vi "SPI API Rack FPGA Modular.vi"() -> ()   [LabVIEW 2014]
uses:
  <userlib>/_NI SPI IP/FPGA/Controllers/Public/Transfer Settings.ctl
  <vilib>/Platform/TimedLoop/XDataNode/timing_clust.ctl
  <vilib>/Platform/TimedLoop/XDataNode/nitl_modes.ctl
  <vilib>/Platform/TimedLoop/XDataNode/wakeup.ctl
  <vilib>/SPI API/SPIAPI/DIO/SPI Digital IO Lines.ctl
  Source/Shared/SPI Utility/CS Bits.ctl
  <vilib>/rvi/Emulation/niFpgaGetClockAttributes.vi
  <vilib>/rvi/Emulation/niFpgaSctlEmulationGetInTimedLoop.vi
  <vilib>/rvi/Emulation/niFpgaEmulationReportErrorSimple.vi
  <vilib>/rvi/Emulation/niFpgaCriticalErrorInLSC.vi
  <vilib>/rvi/interface/RandomDataEmulation/niFpgaRandomDataHandleErrors.vi
  <vilib>/rvi/eio/common/nirviEmuTemplateMethod_errors.vi
  <vilib>/Platform/TimedLoop/XDataNode/XDataNode.xnode
  <vilib>/rvi/DataTransferAndStorage/Container/XNode/niFpgaContainer.xnode
  <vilib>/rvi/interface/RandomDataEmulation/nirviRandomDataFpgaReadWriteTemplate.vi
  <vilib>/eio/EIONode/EIONode.xnode
  <vilib>/Platform/TimedLoop/XDataNode/XDNodeRunTimeDep.lvlib
  Source/Shared/SLSC configuration Shared.lvlib
  <userlib>/_NI SPI IP/FPGA/Controllers/NI SPI IP FPGA.lvlib
panel:
  out "Transfer Length":u8
  out "CS Bit Value":u8
  out "Rack #":u8
  out "read Iterations 3":i32
  out "read Iterations 2":i32
  out "read Iterations 1":i32
  out "FPGA Error":errorcluster
  out "Actual Loop Ticks":u32
  out "oclk div":u32
  out "oclk freq":u32
  in  "Sample Rate (S/s)":u32=10000
  in  "SPI PHY Settings":T1={"Divide Value"=20, "Transfer Length (bits)"=32, "CS Asserted Polarity"=FALSE, "Clock Polarity (CPOL)"=FALSE, "Clock Phase (CPHA)"=FALSE, "Lengthen MISO Setup"=FALSE, "Direction Change Bit"=0, "MOSI Starts as Output"=FALSE, "Tristatable MOSI"=FALSE} {"Direction Change Bit" max=64 step=1; "Transfer Length (bits)" min=1 max=64 step=1}
  out "read Iterations 0":i32
  out "NC":u64
  out "Data to DAC":u64
  out "Chip Select":u8
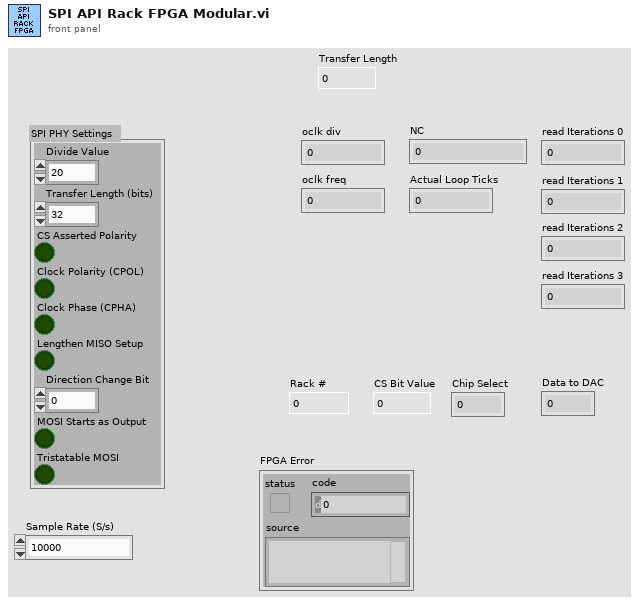
[diagram p1: front panel]
types:
  T1 = typedef "NI SPI IP FPGA.lvlib/Transfer Settings.ctl" = cluster{"Divide Value":u8, "Transfer Length (bits)":u8, "CS Asserted Polarity":bool, "Clock Polarity (CPOL)":bool, "Clock Phase (CPHA)":bool, "Lengthen MISO Setup":bool, "Direction Change Bit":u8, "MOSI Starts as Output":bool, "Tristatable MOSI":bool}
  T2 = typedef "SLSC configuration Shared.lvlib/CS Bits.ctl" = cluster{"CS Bit 1":refnum<k21>, "CS Bit 2":refnum<k21>, "CS Bit 3":refnum<k21>, "CS Bit 4":refnum<k21>}
  T3 = typedef "SPI Digital IO Lines.ctl" = cluster{"SCLK":refnum<k21>, "MISO":refnum<k21>, "MOSI":refnum<k21>, "CS 0":refnum<k21>, "CS 1":refnum<k21>, "CS 2":refnum<k21>, "CS 3":refnum<k21>, "CS 4":refnum<k21>, "CS 5":refnum<k21>}
  T4 = typedef "Internal Data (SPI API).ctl" = cluster{"DLU To SPI Engine Data FIFO":refnum<k21>, "SPI Engine to DLU Data FIFO":refnum<k21>, "Data to SPI Engine (Cache) Register":refnum<k21>, "SPI PHY Settings to SPI Engine (Cahche) Register":refnum<k21>}
  T5 = typedef "XDNodeRunTimeDep.lvlib/timing_clust.ctl" = cluster{"Expected End [f-1]":u64, "Actual End [f-1]":u64, "Finished Late? [f-1]":bool, "Expected End [i-1]":u64, "Actual End [i-1]":u64, "Finished Late? [i-1]":bool, "Expected Start [i]":u64, "Actual Start [i]":u64, "Expected Start [f]":u64, "Actual Start [f]":u64, "Source Name":string, "Structure Name":string, "Period":i64, "Deadline":i64, "Offset":i64, "Start":i64, "Priority":i32, "Timeout":i32, "Mode":T6, "Wakeup Reason":T7, "Error":errorcluster, "Source Type":string, "Secondary Source Type":string, "Global End Time":u64, "Global Start Time":u64, "Frame Duration":u64, "Iteration Duration":u64, "Assigned CPU":i32, "I/O Scan Engine Mode":u32}
  T6 = typedef "XDNodeRunTimeDep.lvlib/nitl_modes.ctl" = enum32{"No Change", "Process missed periods, maintain original phase", "Discard missed periods, maintain original phase", "Process missed periods, ignore original phase", "Discard missed periods, ignore original phase"}
  T7 = typedef "XDNodeRunTimeDep.lvlib/wakeup.ctl" = enum32{"Normal", "Aborted", "Asynchronous wakeup", "Timing source error", "Timed loop error", "Timeout"}
  T8 = typedef "SPI Response Information.ctl" = cluster{"Data to Node":u64, "Node Id":u16}
  T9 = typedef "NI SPI IP FPGA.lvlib/Spi Master Inputs.ctl" = cluster{"MISO":bool}
  T10 = typedef "NI SPI IP FPGA.lvlib/Spi Master Outputs.ctl" = cluster{"Chip Select":bool, "Clock":bool, "MOSI":bool, "MOSI OE":bool}
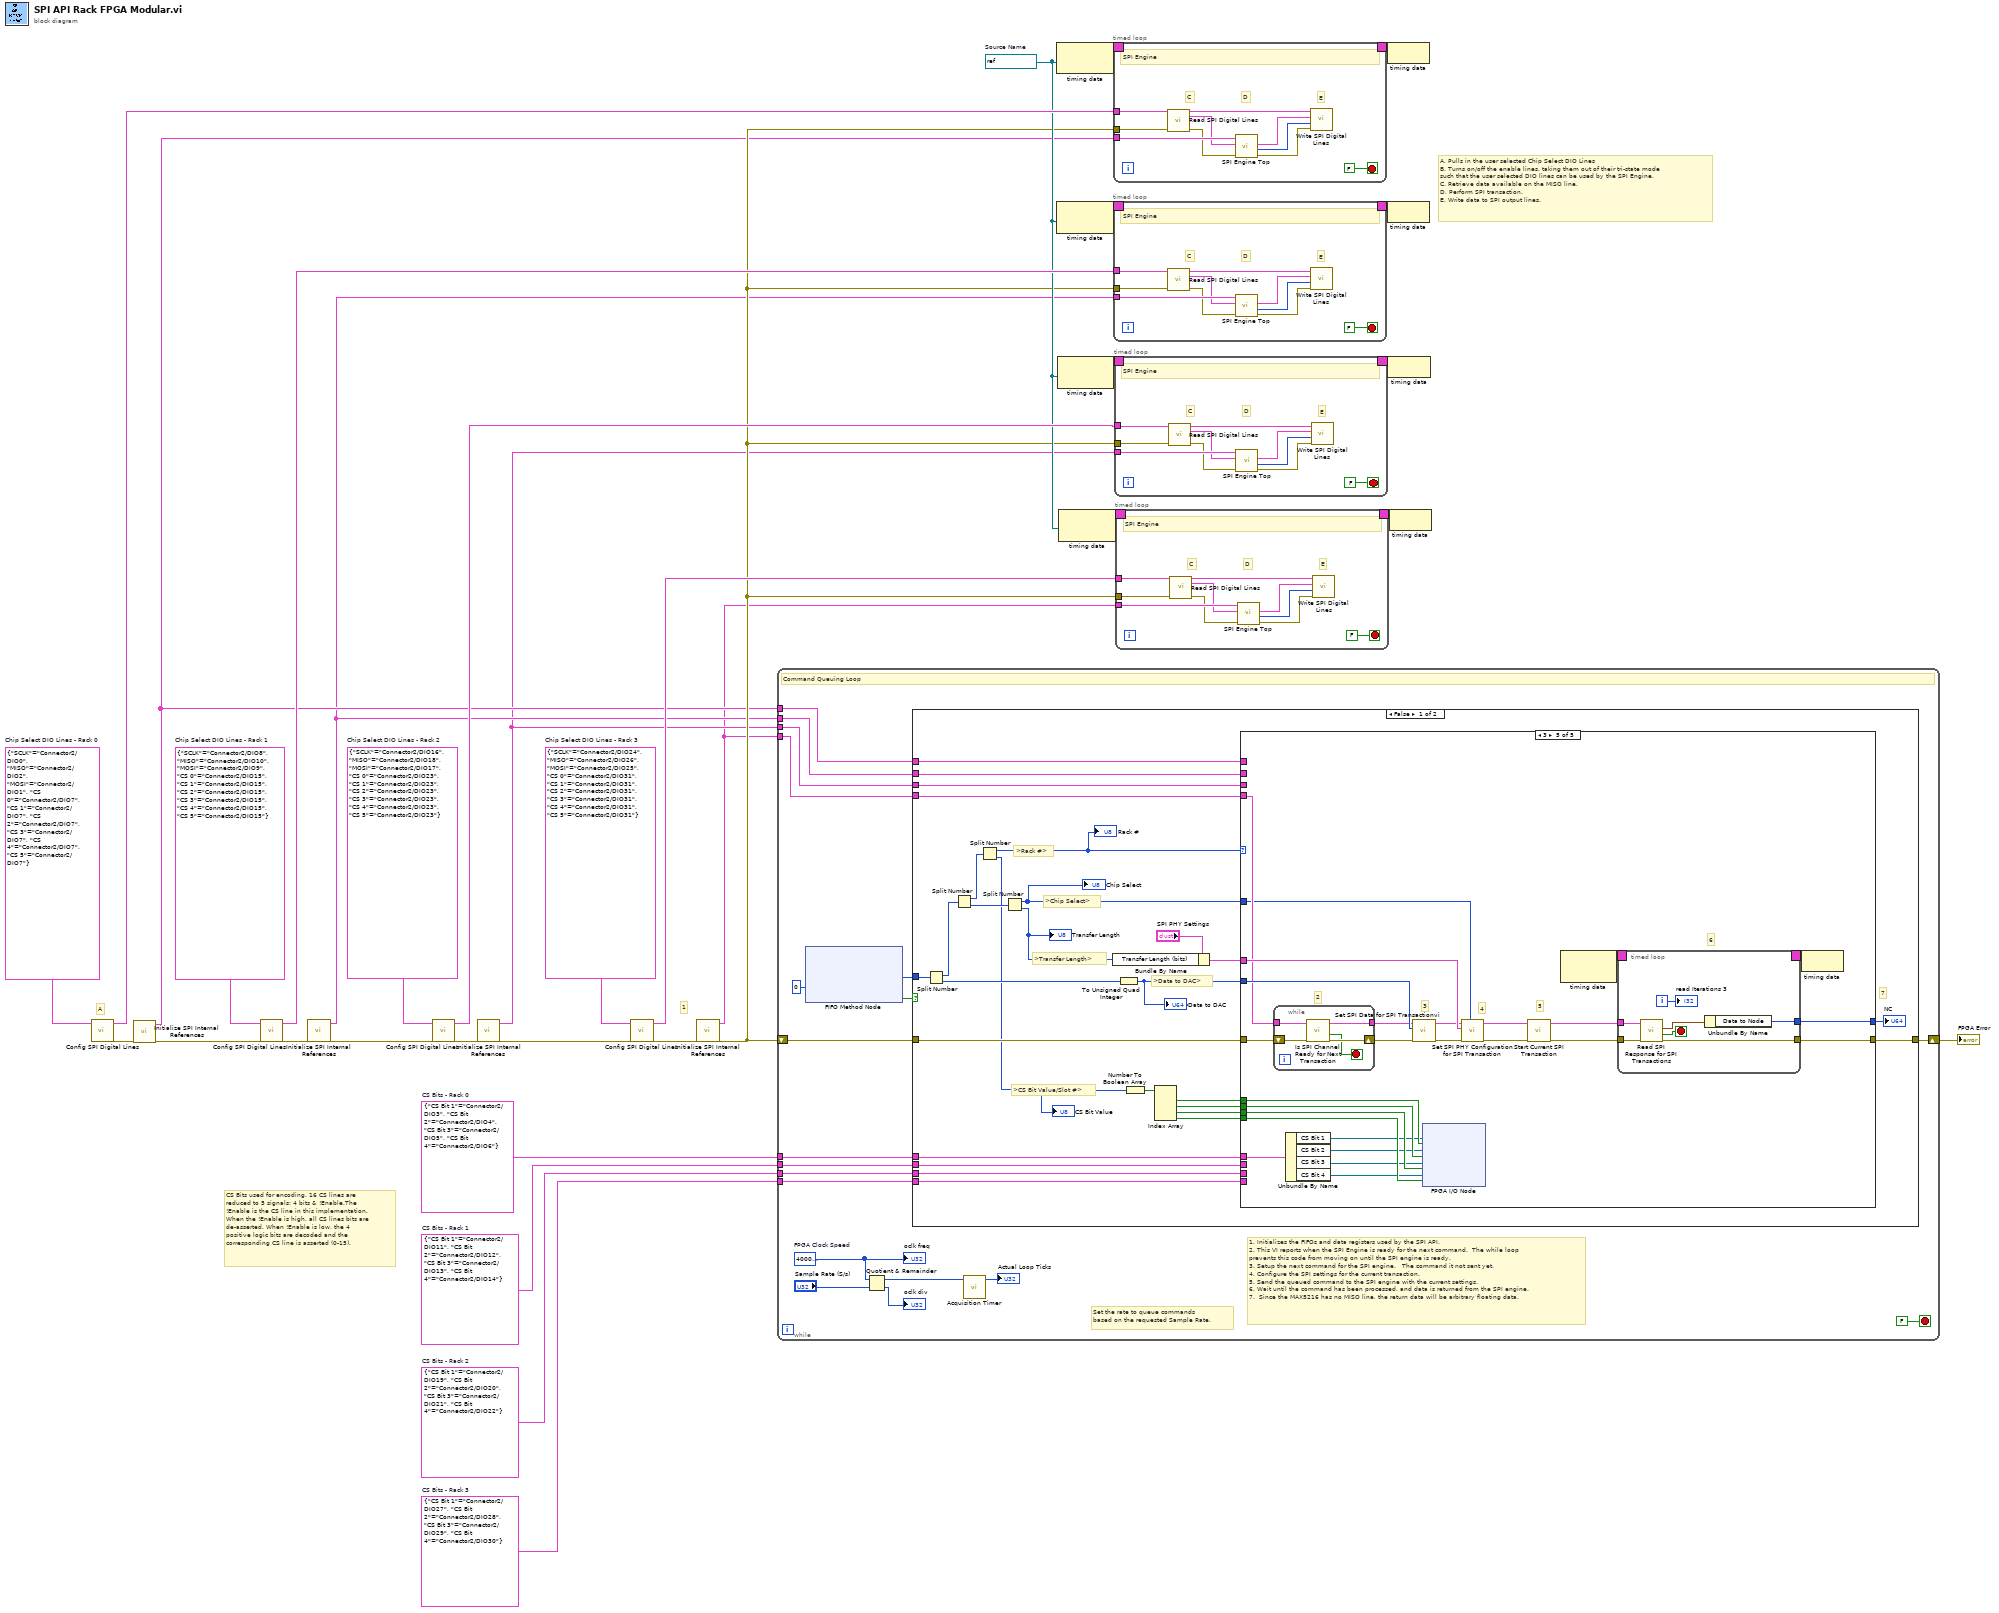
[diagram p0: block diagram]
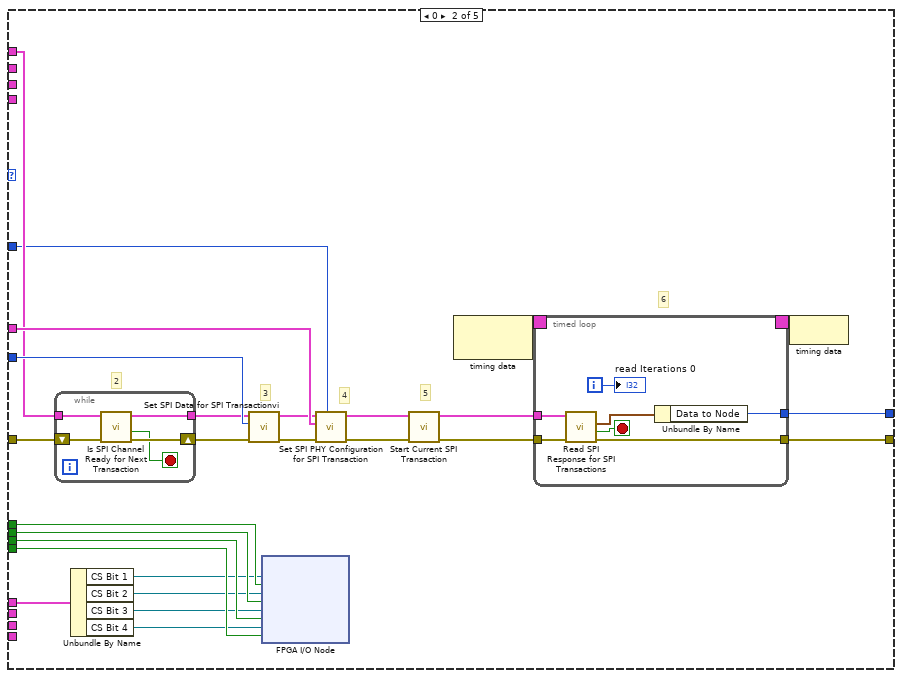
[diagram p3: hidden frame]
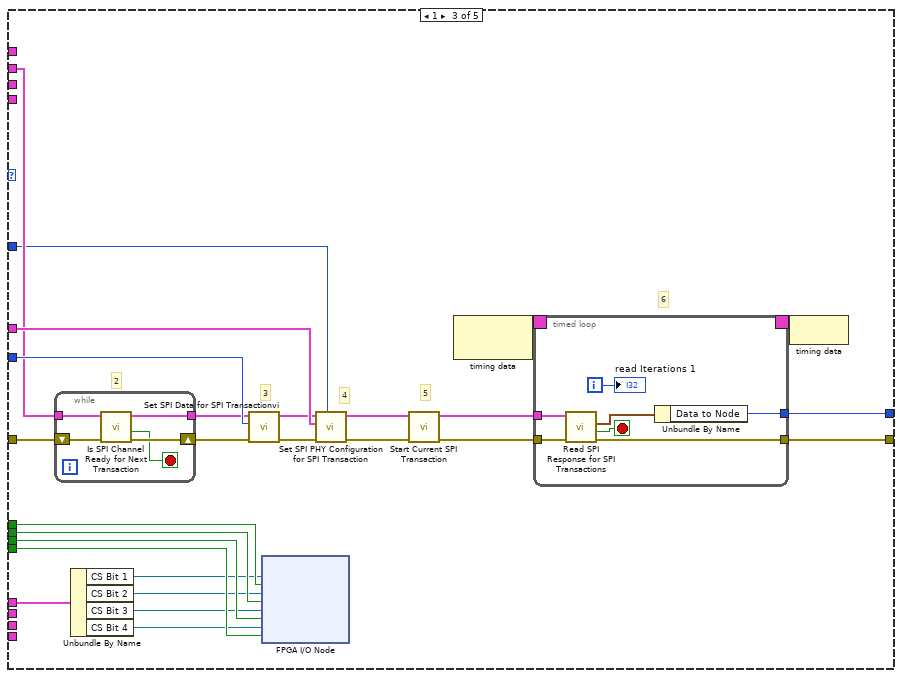
[diagram p4: hidden frame]
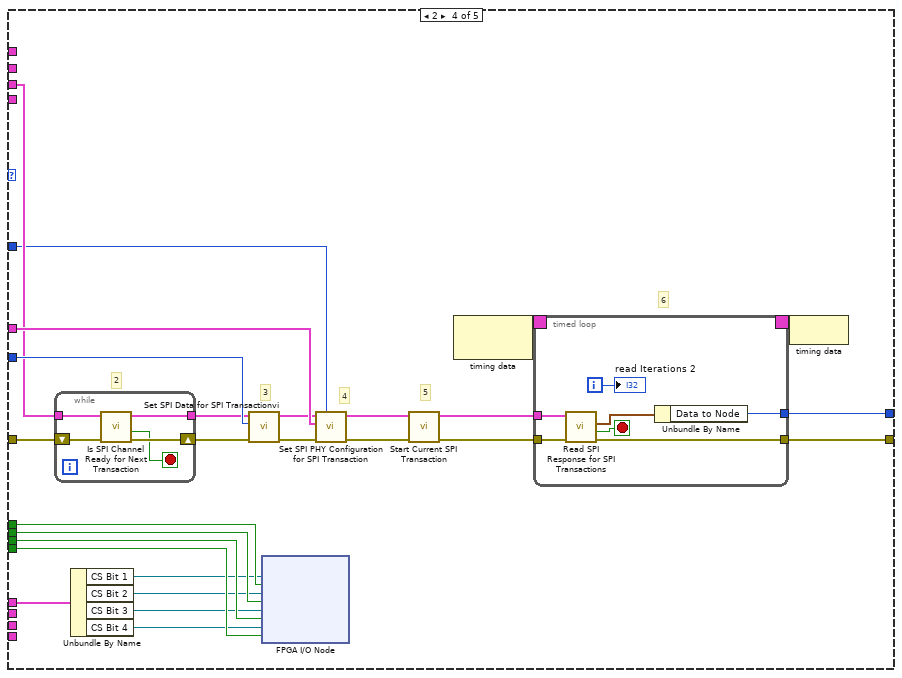
[diagram p5: hidden frame]
diagram:
  w5 = T2 {"CS Bit 1"="Connector2/DIO27", "CS Bit 2"="Connector2/DIO28", "CS Bit 3"="Connector2/DIO29", "CS Bit 4"="Connector2/DIO30"}  # CS Bits - Rack 3
  w6 = T2 {"CS Bit 1"="Connector2/DIO19", "CS Bit 2"="Connector2/DIO20", "CS Bit 3"="Connector2/DIO21", "CS Bit 4"="Connector2/DIO22"}  # CS Bits - Rack 2
  w7 = T2 {"CS Bit 1"="Connector2/DIO11", "CS Bit 2"="Connector2/DIO12", "CS Bit 3"="Connector2/DIO13", "CS Bit 4"="Connector2/DIO14"}  # CS Bits - Rack 1
  w8 = T2 {"CS Bit 1"="Connector2/DIO3", "CS Bit 2"="Connector2/DIO4", "CS Bit 3"="Connector2/DIO5", "CS Bit 4"="Connector2/DIO6"}  # CS Bits - Rack 0
  w21 = T3 {"SCLK"="Connector2/DIO24", "MISO"="Connector2/DIO26", "MOSI"="Connector2/DIO25", "CS 0"="Connector2/DIO31", "CS 1"="Connector2/DIO31", "CS 2"="Connector2/DIO31", "CS 3"="Connector2/DIO31", "CS 4"="Connector2/DIO31", "CS 5"="Connector2/DIO31"}  # Chip Select DIO Lines - Rack 3
  w25 = T3 {"SCLK"="Connector2/DIO16", "MISO"="Connector2/DIO18", "MOSI"="Connector2/DIO17", "CS 0"="Connector2/DIO23", "CS 1"="Connector2/DIO23", "CS 2"="Connector2/DIO23", "CS 3"="Connector2/DIO23", "CS 4"="Connector2/DIO23", "CS 5"="Connector2/DIO23"}  # Chip Select DIO Lines - Rack 2
  w28 = T3 {"SCLK"="Connector2/DIO8", "MISO"="Connector2/DIO10", "MOSI"="Connector2/DIO9", "CS 0"="Connector2/DIO15", "CS 1"="Connector2/DIO15", "CS 2"="Connector2/DIO15", "CS 3"="Connector2/DIO15", "CS 4"="Connector2/DIO15", "CS 5"="Connector2/DIO15"}  # Chip Select DIO Lines - Rack 1
  w32 = T3 {"SCLK"="Connector2/DIO0", "MISO"="Connector2/DIO2", "MOSI"="Connector2/DIO1", "CS 0"="Connector2/DIO7", "CS 1"="Connector2/DIO7", "CS 2"="Connector2/DIO7", "CS 3"="Connector2/DIO7", "CS 4"="Connector2/DIO7", "CS 5"="Connector2/DIO7"}  # Chip Select DIO Lines - Rack 0
  w18 = refnum<k21> "120MHz"  # Source Name
  # "CS Bits used for encoding. 16 CS lines are \nreduced to 5 signals: 4 bits & !Enable.The \n!Enable is the CS line in this implementation.\nWhen the !Enable is high, all CS lines bits are\nde-asserted. When !Enable is low, the 4\npositive logic bits are decoded and the\ncorresponding CS line is asserted (0-15)."
  # "A. Pulls in the user selected Chip Select DIO Lines\nB. Turns on/off the enable lines, taking them out of their tri-state mode \nsuch that the user selected DIO lines can be used by the SPI Engine.\nC. Retrieve data available on the MISO line.\nD. Perform SPI transaction.\nE. Write data to SPI output lines."
  # "A"
  # "1"
  n1 = call <vilib>:"Config SPI Digital Lines.vi"("SPI DIO Lines"=w32) -> ("error out"=w16:errorcluster, "Chip Select DIO Lines"=w27:T3)  [unwired: 9 in]
  n2 = call <vilib>:"Initialize SPI Internal References.vi"("error in"=w16) -> ("error out"=w15:errorcluster, "SPI API References"=w4:T4)  [unwired: 9 in]
  n3 = call <vilib>:"Config SPI Digital Lines.vi"("error in"=w15, "SPI DIO Lines"=w28) -> ("error out"=w14:errorcluster, "Chip Select DIO Lines"=w26:T3)  [unwired: 8 in]
  n4 = call <vilib>:"Initialize SPI Internal References.vi"("error in"=w14) -> ("error out"=w13:errorcluster, "SPI API References"=w3:T4)  [unwired: 9 in]
  n5 = call <vilib>:"Config SPI Digital Lines.vi"("error in"=w13, "SPI DIO Lines"=w25) -> ("error out"=w12:errorcluster, "Chip Select DIO Lines"=w22:T3)  [unwired: 8 in]
  n6 = call <vilib>:"Initialize SPI Internal References.vi"("error in"=w12) -> ("error out"=w11:errorcluster, "SPI API References"=w2:T4)  [unwired: 9 in]
  n7 = call <vilib>:"Config SPI Digital Lines.vi"("error in"=w11, "SPI DIO Lines"=w21) -> ("error out"=w10:errorcluster, "Chip Select DIO Lines"=w17:T3)  [unwired: 8 in]
  n8 = call <vilib>:"Initialize SPI Internal References.vi"("error in"=w10) -> ("error out"=w9:errorcluster, "SPI API References"=w1:T4)  [unwired: 9 in]
  n9 = while {
    shift-right: [w50] -> w31
    shift-left: w9 -> [w52]
    tunnel: w8 -> [w45]
    tunnel: w7 -> [w44]
    tunnel: w6 -> [w43]
    tunnel: w5 -> [w42]
    tunnel: w4 -> [w41]
    tunnel: w3 -> [w38]
    tunnel: w2 -> [w39]
    tunnel: w1 -> [w40]
    stop <- FALSE stop-if-true
    w49 = u32 40000000  # FPGA Clock Speed
    # "1. Initializes the FIFOs and data registers used by the SPI API.\n2. This VI reports when the SPI Engine is ready for the next command.  The while loop \nprevents this code from moving on until the SPI engine is ready.\n3. Setup the next command for the SPI engine.   The command it not sent yet.\n4. Configure the SPI settings for the current transaction.\n5. Send the queued command to the SPI engine with the current settings.\n6. Wait until the command has been processed, and data is returned from the SPI engine.\n7.  Since the MAX5216 has no MISO line, the return data will be arbitrary floating data."
    # "Set the rate to queue commands\nbased on the requested Sample Rate."
    # "Command Queuing Loop"
    n10 = xnode ("FIFO Method Node")("Timeout"=0) -> ("Element"=w37:u64, "Timed Out?"=w36:bool)  [unwired: 1 in, 1 out]
    n11 = Quotient & Remainder(x=w49, y="Sample Rate (S/s)") -> (x-y*floor(x/y)=w46:u32, floor(x/y)=→"oclk div":u32)
    n12 = case shown="False" w36 {
      tunnel: w52 -> [w81 w251]
      tunnel: [w80 w251] -> w50
      tunnel: w37 -> [w78 _]
      tunnel: w45 -> [w65 _]
      tunnel: w44 -> [w64 _]
      tunnel: w43 -> [w63 _]
      tunnel: w42 -> [w62 _]
      tunnel: w41 -> [w61 _]
      tunnel: w40 -> [w60 _]
      tunnel: w39 -> [w59 _]
      tunnel: w38 -> [w58 _]
      frame False {
        # ">Transfer Length>"
        # ">CS Bit Value/Slot #>"
        # ">Rack #>"
        # ">Data to DAC>"
        # ">Chip Select>"
        # "7"
        n13 = Split Number(x=w78) -> (hi(x)=w76:u32, lo(x)=w77:u32)
        n14 = Split Number(x=w76) -> (hi(x)=w57:u16, lo(x)=w75:u16)
        n15 = Split Number(x=w57) -> (hi(x)=w55:u8, lo(x)=w54:u8)
        "Rack #" <- w55
        "CS Bit Value" <- w54
        n16 = Split Number(x=w75) -> (hi(x)=w56:u8, lo(x)=w72:u8)
        "Chip Select" <- w56
        "Transfer Length" <- w72
        n17 = Bundle By Name(cluster="SPI PHY Settings", "Transfer Length (bits)"=w72) -> (w73:T1)
        n18 = To Unsigned Quad Integer(1:w77) -> (0:w71:u64)
        "Data to DAC" <- w71
        n19 = Number To Boolean Array(number=w54) -> (Boolean array=w70:bool[])
        n20 = Index Array(array=w70) -> (element #1=w69:bool, element #2=w68:bool, element #3=w67:bool, element #4=w66:bool)  [unwired: 4 in]
        n21 = case shown="3" w55 {
          tunnel: w81 -> [w82 w106 w148 w190 w232]
          tunnel: [w82 w105 w147 w189 w231] -> w80
          tunnel: [_ w104 w146 w188 w230] -> w79
          tunnel: w73 -> [_ w103 w145 w187 w229]
          tunnel: w71 -> [_ w102 w144 w186 w228]
          tunnel: w69 -> [_ w101 w143 w185 w227]
          tunnel: w68 -> [_ w100 w142 w184 w226]
          tunnel: w67 -> [_ w99 w141 w183 w225]
          tunnel: w66 -> [_ w98 w140 w182 w224]
          tunnel: w65 -> [_ w97 w139 w181 w223]
          tunnel: w64 -> [_ _ _ _ _]
          tunnel: w63 -> [_ _ _ _ _]
          tunnel: w62 -> [_ _ _ _ _]
          tunnel: w61 -> [_ w84 _ _ _]
          tunnel: w60 -> [_ _ _ _ w210]
          tunnel: w59 -> [_ _ _ w168 _]
          tunnel: w58 -> [_ _ w126 _ _]
          tunnel: w56 -> [_ w83 w125 w167 w209]
          frame Default {
          }
          frame 0 {
            # "6"
            # "5"
            # "4"
            # "3"
            # "2"
            n22 = while {
              shift-right: [w113] -> w96
              shift-left: w106 -> [w111]
              tunnel: w84 -> [w109]
              tunnel: [w112] -> w95
              stop <- w110 stop-if-true
              n23 = call <vilib>:"Is SPI Channel Ready for Next Transaction.vi"("error in"=w111, "Private Data In"=w109) -> ("error out"=w113:errorcluster, "SPI Channel Ready"=w110:bool, "Private Data Out"=w112:T4)  [unwired: 6 in, 1 out]
            }
            n24 = Unbundle By Name(w97) -> ("CS Bit 1"=w88:refnum<k21>, "CS Bit 2"=w87:refnum<k21>, "CS Bit 3"=w86:refnum<k21>, "CS Bit 4"=w85:refnum<k21>)
            n25 = call <vilib>:"Set SPI Data for SPI Transactionvi.vi"("error in"=w96, "Data In"=w102, "Private Data In"=w95) -> ("error out"=w92:errorcluster, "Private Data Out"=w93:T4)  [unwired: 7 in]
            n26 = xnode "FPGA I/O Node"("I/O Item"=w101, "FPGA I/O In"=w88, "I/O Item"=w100, "FPGA I/O In"=w87, "I/O Item"=w99, "FPGA I/O In"=w86, "I/O Item"=w98, "FPGA I/O In"=w85) -> ()  [unwired: 4 out]
            n27 = call <vilib>:"Set SPI PHY Configuration for SPI Transaction.vi"("Chip Select"=w83, "error in"=w92, "SPI PHY Settings"=w103, "Private Data In"=w93) -> ("error out"=w90:errorcluster, "Private Data Out"=w91:T4)  [unwired: 6 in]
            n28 = call <vilib>:"Start Current SPI Transaction.vi"("error in"=w90, "Private Data In"=w91) -> ("error out"=w94:errorcluster, "Private Data Out"=w89:T4)  [unwired: 7 in, 1 out]
            n29 = node-c288() -> (w108:T5)  [unwired: 1 in]
            n30 = timed-loop {
              timing: w108 -> [_]
              timing-out: [_] -> w107
              tunnel: w94 -> [w120]
              tunnel: w89 -> [w119]
              tunnel: [w114] -> w104
              tunnel: [w116] -> w105
              i -> [w115]
              stop <- w118 stop-if-true
              n31 = call <vilib>:"Read SPI Response for SPI Transactions.vi"("error in"=w120, "Private Data In"=w119) -> ("error out"=w116:errorcluster, "Read Data Valid?"=w118:bool, "Read Data"=w117:T8)  [unwired: 6 in, 1 out]
              n32 = Unbundle By Name(w117) -> ("Data to Node"=w114:u64)
              "read Iterations 0" <- w115
            }
            n33 = node-c288(w107) -> ()
          }
          frame 1 {
            # "6"
            # "5"
            # "4"
            # "3"
            # "2"
            n34 = while {
              shift-right: [w155] -> w138
              shift-left: w148 -> [w153]
              tunnel: w126 -> [w151]
              tunnel: [w154] -> w137
              stop <- w152 stop-if-true
              n35 = call <vilib>:"Is SPI Channel Ready for Next Transaction.vi"("error in"=w153, "Private Data In"=w151) -> ("error out"=w155:errorcluster, "SPI Channel Ready"=w152:bool, "Private Data Out"=w154:T4)  [unwired: 6 in, 1 out]
            }
            n36 = Unbundle By Name(w139) -> ("CS Bit 1"=w130:refnum<k21>, "CS Bit 2"=w129:refnum<k21>, "CS Bit 3"=w128:refnum<k21>, "CS Bit 4"=w127:refnum<k21>)
            n37 = call <vilib>:"Set SPI Data for SPI Transactionvi.vi"("error in"=w138, "Data In"=w144, "Private Data In"=w137) -> ("error out"=w134:errorcluster, "Private Data Out"=w135:T4)  [unwired: 7 in]
            n38 = xnode "FPGA I/O Node"("I/O Item"=w143, "FPGA I/O In"=w130, "I/O Item"=w142, "FPGA I/O In"=w129, "I/O Item"=w141, "FPGA I/O In"=w128, "I/O Item"=w140, "FPGA I/O In"=w127) -> ()  [unwired: 4 out]
            n39 = call <vilib>:"Set SPI PHY Configuration for SPI Transaction.vi"("Chip Select"=w125, "error in"=w134, "SPI PHY Settings"=w145, "Private Data In"=w135) -> ("error out"=w132:errorcluster, "Private Data Out"=w133:T4)  [unwired: 6 in]
            n40 = call <vilib>:"Start Current SPI Transaction.vi"("error in"=w132, "Private Data In"=w133) -> ("error out"=w136:errorcluster, "Private Data Out"=w131:T4)  [unwired: 7 in, 1 out]
            n41 = node-c288() -> (w150:T5)  [unwired: 1 in]
            n42 = timed-loop {
              timing: w150 -> [_]
              timing-out: [_] -> w149
              tunnel: w136 -> [w162]
              tunnel: w131 -> [w161]
              tunnel: [w156] -> w146
              tunnel: [w158] -> w147
              i -> [w157]
              stop <- w160 stop-if-true
              n43 = call <vilib>:"Read SPI Response for SPI Transactions.vi"("error in"=w162, "Private Data In"=w161) -> ("error out"=w158:errorcluster, "Read Data Valid?"=w160:bool, "Read Data"=w159:T8)  [unwired: 6 in, 1 out]
              n44 = Unbundle By Name(w159) -> ("Data to Node"=w156:u64)
              "read Iterations 1" <- w157
            }
            n45 = node-c288(w149) -> ()
          }
          frame 2 {
            # "6"
            # "5"
            # "4"
            # "3"
            # "2"
            n46 = while {
              shift-right: [w197] -> w180
              shift-left: w190 -> [w195]
              tunnel: w168 -> [w193]
              tunnel: [w196] -> w179
              stop <- w194 stop-if-true
              n47 = call <vilib>:"Is SPI Channel Ready for Next Transaction.vi"("error in"=w195, "Private Data In"=w193) -> ("error out"=w197:errorcluster, "SPI Channel Ready"=w194:bool, "Private Data Out"=w196:T4)  [unwired: 6 in, 1 out]
            }
            n48 = Unbundle By Name(w181) -> ("CS Bit 1"=w172:refnum<k21>, "CS Bit 2"=w171:refnum<k21>, "CS Bit 3"=w170:refnum<k21>, "CS Bit 4"=w169:refnum<k21>)
            n49 = call <vilib>:"Set SPI Data for SPI Transactionvi.vi"("error in"=w180, "Data In"=w186, "Private Data In"=w179) -> ("error out"=w176:errorcluster, "Private Data Out"=w177:T4)  [unwired: 7 in]
            n50 = xnode "FPGA I/O Node"("I/O Item"=w185, "FPGA I/O In"=w172, "I/O Item"=w184, "FPGA I/O In"=w171, "I/O Item"=w183, "FPGA I/O In"=w170, "I/O Item"=w182, "FPGA I/O In"=w169) -> ()  [unwired: 4 out]
            n51 = call <vilib>:"Set SPI PHY Configuration for SPI Transaction.vi"("Chip Select"=w167, "error in"=w176, "SPI PHY Settings"=w187, "Private Data In"=w177) -> ("error out"=w174:errorcluster, "Private Data Out"=w175:T4)  [unwired: 6 in]
            n52 = call <vilib>:"Start Current SPI Transaction.vi"("error in"=w174, "Private Data In"=w175) -> ("error out"=w178:errorcluster, "Private Data Out"=w173:T4)  [unwired: 7 in, 1 out]
            n53 = node-c288() -> (w192:T5)  [unwired: 1 in]
            n54 = timed-loop {
              timing: w192 -> [_]
              timing-out: [_] -> w191
              tunnel: w178 -> [w204]
              tunnel: w173 -> [w203]
              tunnel: [w198] -> w188
              tunnel: [w200] -> w189
              i -> [w199]
              stop <- w202 stop-if-true
              n55 = call <vilib>:"Read SPI Response for SPI Transactions.vi"("error in"=w204, "Private Data In"=w203) -> ("error out"=w200:errorcluster, "Read Data Valid?"=w202:bool, "Read Data"=w201:T8)  [unwired: 6 in, 1 out]
              n56 = Unbundle By Name(w201) -> ("Data to Node"=w198:u64)
              "read Iterations 2" <- w199
            }
            n57 = node-c288(w191) -> ()
          }
          frame 3 {
            # "6"
            # "5"
            # "4"
            # "3"
            # "2"
            n58 = while {
              shift-right: [w239] -> w222
              shift-left: w232 -> [w237]
              tunnel: w210 -> [w235]
              tunnel: [w238] -> w221
              stop <- w236 stop-if-true
              n59 = call <vilib>:"Is SPI Channel Ready for Next Transaction.vi"("error in"=w237, "Private Data In"=w235) -> ("error out"=w239:errorcluster, "SPI Channel Ready"=w236:bool, "Private Data Out"=w238:T4)  [unwired: 6 in, 1 out]
            }
            n60 = Unbundle By Name(w223) -> ("CS Bit 1"=w214:refnum<k21>, "CS Bit 2"=w213:refnum<k21>, "CS Bit 3"=w212:refnum<k21>, "CS Bit 4"=w211:refnum<k21>)
            n61 = call <vilib>:"Set SPI Data for SPI Transactionvi.vi"("error in"=w222, "Data In"=w228, "Private Data In"=w221) -> ("error out"=w218:errorcluster, "Private Data Out"=w219:T4)  [unwired: 7 in]
            n62 = xnode "FPGA I/O Node"("I/O Item"=w227, "FPGA I/O In"=w214, "I/O Item"=w226, "FPGA I/O In"=w213, "I/O Item"=w225, "FPGA I/O In"=w212, "I/O Item"=w224, "FPGA I/O In"=w211) -> ()  [unwired: 4 out]
            n63 = call <vilib>:"Set SPI PHY Configuration for SPI Transaction.vi"("Chip Select"=w209, "error in"=w218, "SPI PHY Settings"=w229, "Private Data In"=w219) -> ("error out"=w216:errorcluster, "Private Data Out"=w217:T4)  [unwired: 6 in]
            n64 = call <vilib>:"Start Current SPI Transaction.vi"("error in"=w216, "Private Data In"=w217) -> ("error out"=w220:errorcluster, "Private Data Out"=w215:T4)  [unwired: 7 in, 1 out]
            n65 = node-c288() -> (w234:T5)  [unwired: 1 in]
            n66 = timed-loop {
              timing: w234 -> [_]
              timing-out: [_] -> w233
              tunnel: w220 -> [w246]
              tunnel: w215 -> [w245]
              tunnel: [w240] -> w230
              tunnel: [w242] -> w231
              i -> [w241]
              stop <- w244 stop-if-true
              n67 = call <vilib>:"Read SPI Response for SPI Transactions.vi"("error in"=w246, "Private Data In"=w245) -> ("error out"=w242:errorcluster, "Read Data Valid?"=w244:bool, "Read Data"=w243:T8)  [unwired: 6 in, 1 out]
              n68 = Unbundle By Name(w243) -> ("Data to Node"=w240:u64)
              "read Iterations 3" <- w241
            }
            n69 = node-c288(w233) -> ()
          }
        }
        "NC" <- w79
      }
      frame True {
      }
    }
    n70 = call <vilib>:"Acquisition Timer.vi"("Loop Time (Ticks)"=w46) -> ("Actual Time (Ticks)"=→"Actual Loop Ticks":u32)  [unwired: 10 in]
    "oclk freq" <- w49
  }
  "FPGA Error" <- w31
  n71 = node-c288(w18) -> (w34:T5)
  n72 = node-c288(w18) -> (w30:T5)
  n73 = node-c288(w18) -> (w24:T5)
  n74 = node-c288(w18) -> (w20:T5)
  n75 = timed-loop {
    tunnel: w4 -> [w258]
    tunnel: w9 -> [w256]
    tunnel: w27 -> [w260]
    timing: w34 -> [_]
    timing-out: [_] -> w33
    stop <- FALSE stop-if-true
    # "E"
    # "D"
    # "C"
    # "SPI Engine"
    n76 = call <vilib>:"Read SPI Digital Lines.vi"("Chip Select DIO Lines"=w260, "error in"=w256) -> ("Chip Select DIO Lines Out"=w261:T3, "SPI Read Data"=w257:T9, "error out"=w255:errorcluster)  [unwired: 11 in]
    n77 = call <vilib>:"SPI Engine Top.vi"("error in"=w255, "SPI Read Data"=w257, "SPI API References"=w258) -> ("error out"=w254:errorcluster, "Chip Select ID"=w253:u8, "SPI DIO Output"=w259:T10)  [unwired: 5 in, 1 out]
    n78 = call <vilib>:"Write SPI Digital Lines.vi"("error in"=w254, "CS Index"=w253, "spi output"=w259, "Chip Select DIO Lines"=w261) -> ()  [unwired: 6 in, 2 out]
  }
  n79 = timed-loop {
    tunnel: w3 -> [w270]
    tunnel: w9 -> [w268]
    tunnel: w26 -> [w272]
    timing: w30 -> [_]
    timing-out: [_] -> w29
    stop <- FALSE stop-if-true
    # "E"
    # "D"
    # "C"
    # "SPI Engine"
    n80 = call <vilib>:"Read SPI Digital Lines.vi"("Chip Select DIO Lines"=w272, "error in"=w268) -> ("Chip Select DIO Lines Out"=w273:T3, "SPI Read Data"=w269:T9, "error out"=w267:errorcluster)  [unwired: 11 in]
    n81 = call <vilib>:"SPI Engine Top.vi"("error in"=w267, "SPI Read Data"=w269, "SPI API References"=w270) -> ("error out"=w266:errorcluster, "Chip Select ID"=w265:u8, "SPI DIO Output"=w271:T10)  [unwired: 5 in, 1 out]
    n82 = call <vilib>:"Write SPI Digital Lines.vi"("error in"=w266, "CS Index"=w265, "spi output"=w271, "Chip Select DIO Lines"=w273) -> ()  [unwired: 6 in, 2 out]
  }
  n83 = timed-loop {
    tunnel: w2 -> [w282]
    tunnel: w9 -> [w280]
    tunnel: w22 -> [w284]
    timing: w24 -> [_]
    timing-out: [_] -> w23
    stop <- FALSE stop-if-true
    # "E"
    # "D"
    # "C"
    # "SPI Engine"
    n84 = call <vilib>:"Read SPI Digital Lines.vi"("Chip Select DIO Lines"=w284, "error in"=w280) -> ("Chip Select DIO Lines Out"=w285:T3, "SPI Read Data"=w281:T9, "error out"=w279:errorcluster)  [unwired: 11 in]
    n85 = call <vilib>:"SPI Engine Top.vi"("error in"=w279, "SPI Read Data"=w281, "SPI API References"=w282) -> ("error out"=w278:errorcluster, "Chip Select ID"=w277:u8, "SPI DIO Output"=w283:T10)  [unwired: 5 in, 1 out]
    n86 = call <vilib>:"Write SPI Digital Lines.vi"("error in"=w278, "CS Index"=w277, "spi output"=w283, "Chip Select DIO Lines"=w285) -> ()  [unwired: 6 in, 2 out]
  }
  n87 = timed-loop {
    tunnel: w1 -> [w294]
    tunnel: w9 -> [w292]
    tunnel: w17 -> [w296]
    timing: w20 -> [_]
    timing-out: [_] -> w19
    stop <- FALSE stop-if-true
    # "E"
    # "D"
    # "C"
    # "SPI Engine"
    n88 = call <vilib>:"Read SPI Digital Lines.vi"("Chip Select DIO Lines"=w296, "error in"=w292) -> ("Chip Select DIO Lines Out"=w297:T3, "SPI Read Data"=w293:T9, "error out"=w291:errorcluster)  [unwired: 11 in]
    n89 = call <vilib>:"SPI Engine Top.vi"("error in"=w291, "SPI Read Data"=w293, "SPI API References"=w294) -> ("error out"=w290:errorcluster, "Chip Select ID"=w289:u8, "SPI DIO Output"=w295:T10)  [unwired: 5 in, 1 out]
    n90 = call <vilib>:"Write SPI Digital Lines.vi"("error in"=w290, "CS Index"=w289, "spi output"=w295, "Chip Select DIO Lines"=w297) -> ()  [unwired: 6 in, 2 out]
  }
  n91 = node-c288(w33) -> ()
  n92 = node-c288(w29) -> ()
  n93 = node-c288(w23) -> ()
  n94 = node-c288(w19) -> ()
